vi "Configure Average.vi"(7 "Average On":bool, 8 "error in (no error)":errorcluster, 10 "Number of Averages":i32, 11 "VNA-PNA in":refnum<class "VNA-PNA.lvclass">) -> (0 "error out":errorcluster, 3 "VNA-PNA out":refnum<class "VNA-PNA.lvclass">)   [LabVIEW 2020, in "VNA-PNA.lvclass"]
doc: "Configures the average to use for the sweep"
uses:
  VNA-PNA.lvclass
  C:/Sandbox/Git_Sandbox/WiSpry Test Framework source code (LV20)/WiSpry Test Framework/Instruments/Instrument.lvclass
  C:/Sandbox/Git_Sandbox/WiSpry Test Framework source code (LV20)/WiSpry Test Framework/Instruments/Vector Network Analyzer/Vector Network Analyzer.lvclass
  Instrument.lvclass/Instrument.ctl
  Vector Network Analyzer.lvclass/Vector Network Analyzer.ctl
  Instrument.lvclass
  Vector Network Analyzer.lvclass
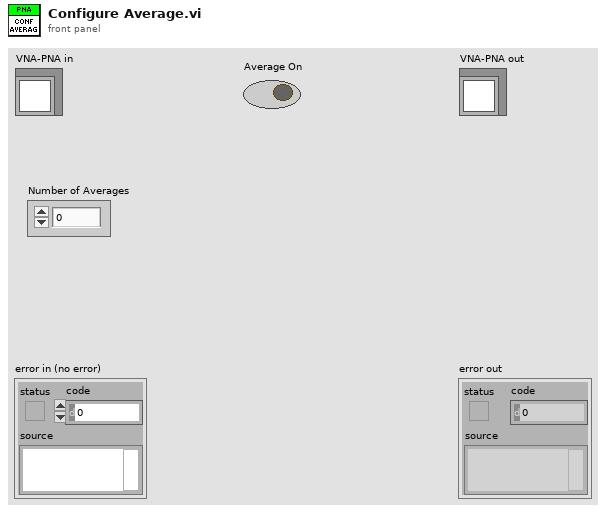
[diagram p1: front panel]
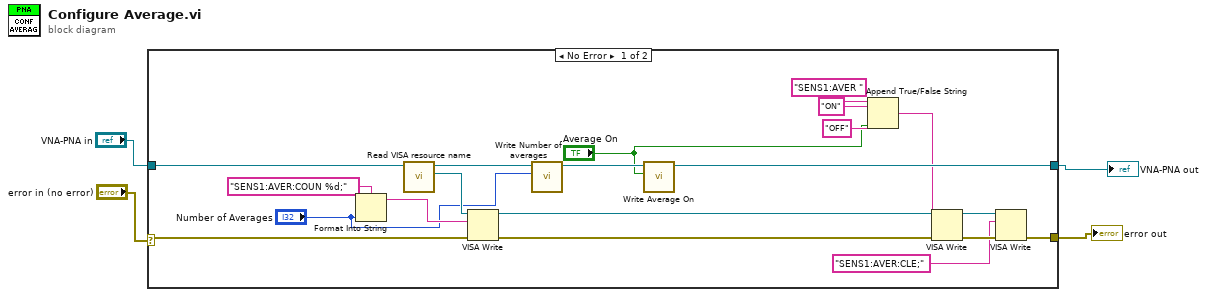
[diagram p0: block diagram]
diagram:
  n1 = case shown="No Error" "error in (no error)" {
    selector: "error in (no error)" -> [w22 w25]
    tunnel: "VNA-PNA in" -> [w23 w26]
    tunnel: [w15 w26] -> w2
    tunnel: [w8 w25] -> w1
    frame No Error {
      n2 = Format Into String(format string="SENS1:AVER:COUN %d;", "Number of Averages") -> (resulting string=w20:string)  [unwired: 2 in, 1 out]
      n3 = call "Read VISA resource name.vi"("Instrument in"=w23) -> ("VISA resource name"=w21:refnum<visa-resource-name>, "Instrument out"=w17:refnum<class "VNA-PNA.lvclass">)  [unwired: 9 in]
      n4 = VISA Write(VISA resource name=w21, write buffer=w20, error in (no error)=w22) -> (VISA resource name out=w10:refnum<visa-resource-name>, error out=w11:errorcluster)  [unwired: 1 out]
      n5 = call "Write Number of averages.vi"("Number of averages"="Number of Averages", "Vector Network Analyzer in"=w17) -> ("Vector Network Analyzer out"=w16:refnum<class "VNA-PNA.lvclass">)  [unwired: 9 in]
      n6 = call "Write Average On.vi"("Average On"="Average On", "Vector Network Analyzer in"=w16) -> ("Vector Network Analyzer out"=w15:refnum<class "VNA-PNA.lvclass">)  [unwired: 9 in]
      n7 = Append True/False String(1:"Average On", 2:"OFF" ("false string"), 3:"ON" ("true string"), 4:"SENS1:AVER " ("string (\"\")")) -> (0:w9:string)
      n8 = VISA Write(VISA resource name=w10, write buffer=w9, error in (no error)=w11) -> (VISA resource name out=w6:refnum<visa-resource-name>, error out=w7:errorcluster)  [unwired: 1 out]
      n9 = VISA Write(VISA resource name=w6, write buffer="SENS1:AVER:CLE;" ("string"), error in (no error)=w7) -> (error out=w8:errorcluster)  [unwired: 2 out]
    }
    frame Error {
    }
  }
  "error out" <- w1
  "VNA-PNA out" <- w2
